vi "Settings_Load.vi"(8 "error in":errorcluster) -> (0 "error out":errorcluster, 3 "DataCluster out":T1)   [LabVIEW 2020]
uses:
  DataCluster.ctl
  <vilib>/Utility/xml.llb/Read From XML File(string).vi
panel:
  in  "DefaultValues":T1={"Core"={"Current VI Reference"=refnum, "Close Panel on Exit?"=FALSE, "Exit"=FALSE}, "Connections"={"Arduino"={"VISA"="Sample", "Data Feed"="", "Connected"=FALSE}, "Ready"=FALSE}, "Files"={"Path"=path "", "Filename"="", "File List"=0, "Buffer"={"Buffer"=refnum, "Size"=0}, "Downloading"=FALSE}}
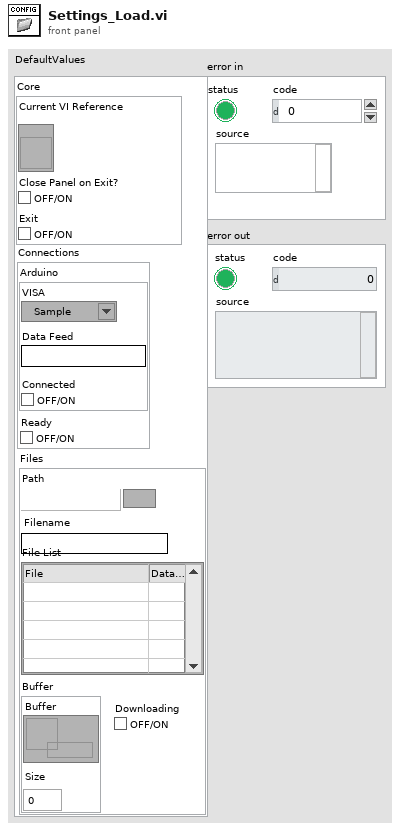
[diagram p1: front panel]
types:
  T1 = typedef "DataCluster.ctl" = cluster{"Core":cluster{"Current VI Reference":refnum<vi>, "Close Panel on Exit?":bool, "Exit":bool}, "Connections":cluster{"Arduino":cluster{"VISA":refnum<visa-resource-name>, "Data Feed":string, "Connected":bool}, "Ready":bool}, "Files":cluster{"Path":path, "Filename":string, "File List":i32, "Buffer":cluster{"Buffer":refnum<queue>, "Size":i32}, "Downloading":bool}}
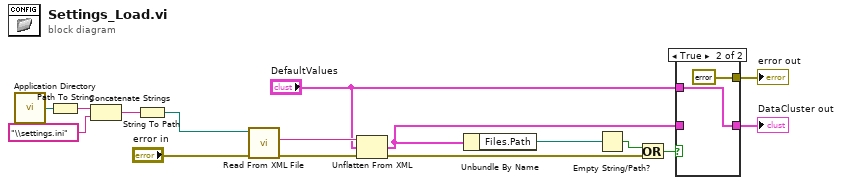
[diagram p0: block diagram]
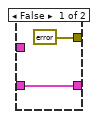
[diagram p2: hidden frame]
diagram:
  n1 = call <vilib>:"Application Directory.vi"() -> ("Application Directory"=w15:path)
  n2 = Path To String(path=w15) -> (string=w16:string)
  n3 = Concatenate Strings(w16, "\\settings.ini" ("string")) -> (w13:string)
  n4 = String To Path(string=w13) -> (path=w11:path)
  n5 = call-poly <vilib>:"Read From XML File.vi"("error in (no error)"="error in", "XML File Path"=w11) -> ("error out"=w9:errorcluster, "XML Elements"=w10:string)  [unwired: 7 in, 1 out]
  n6 = Unflatten From XML(xml string=w10, type="DefaultValues", error in (no error)=w9) -> (value=w7:T1, error out=w5:errorcluster)
  n7 = Unbundle By Name(w7) -> ("Files.Path"=w1:path)
  n8 = Empty String/Path?(string/path=w1) -> (empty?=w2:bool)
  n9 = Or(x=w2, y=w5) -> (x .or. y?=w6:bool)
  n10 = case shown="True" w6 {
    tunnel: [w18 w20] -> w8
    tunnel: "DefaultValues" -> [_ w20]
    tunnel: w7 -> [w18 _]
    tunnel: [errorcluster {"status"=FALSE, "code"=0, "source"=""} ("error in") errorcluster {"status"=FALSE, "code"=0, "source"=""} ("error in")] -> w3
    frame False {
    }
    frame True {
    }
  }
  "error out" <- w3
  "DataCluster out" <- w8
